vi "Clock Array to Clock Map.vi"(8 "error in (no error)":errorcluster, 10 "Clock Conversion Array":T3[](array[typedef]), 11 "Clock Convert Map in":T1) -> (0 "error out":errorcluster, 3 "Clock Convert Map out":T1)   [LabVIEW 2021, in "CIFClocks.lvlib"]
uses:
  CIFClocks.lvlib
  Typedef/Clock Conversion Map.ctl
  Typedef/Timestamp Pair.ctl
  Typedef/Clock Conversion.ctl
  <vilib>/Utility/miscctls.llb/LVMapReplaceAction.ctl
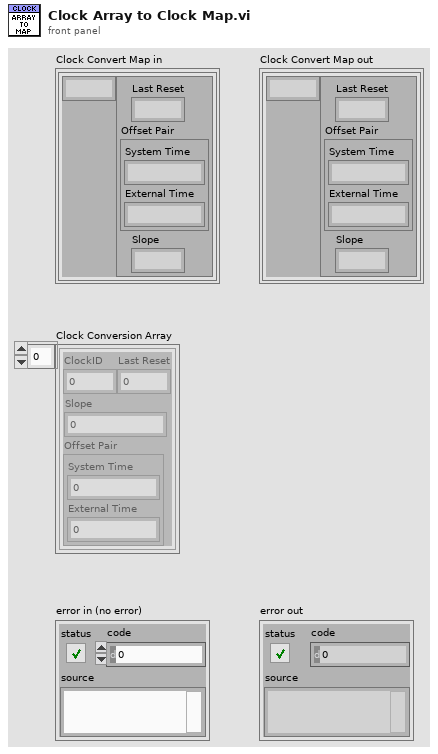
[diagram p1: front panel]
types:
  T1 = typedef "CIFClocks.lvlib/Clock Conversion Map.ctl" = map{u8, cluster{"Last Reset":u64, "Offset Pair":T2, "Slope":dbl}}
  T2 = typedef "CIFClocks.lvlib/Timestamp Pair.ctl" = cluster{"System Time":i64, "External Time":i64}
  T3 = typedef "CIFClocks.lvlib/Clock Conversion.ctl" = cluster{"ClockID":u8, "Last Reset":u64, "Offset Pair":T2, "Slope":dbl}
  T4 = typedef "LVMapReplaceAction.ctl" = enum32{"Modify Entry only if found", "Add or Modify Entry", "Delete Entry"}
  T5 = cluster{"Last Reset":u64, "Offset Pair":T2, "Slope":dbl}
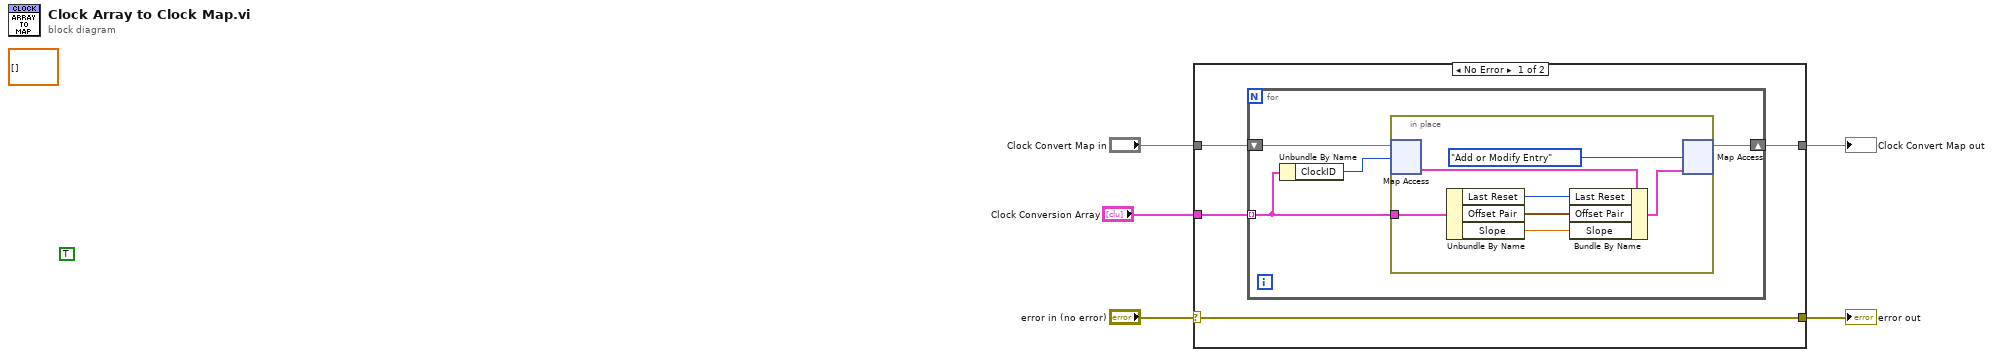
[diagram p0: block diagram]
diagram:
  (unwired) TRUE
  (unwired) dbl[][] []
  n1 = case shown="No Error" "error in (no error)" {
    selector: "error in (no error)" -> [w9 w22]
    tunnel: "Clock Convert Map in" -> [w8 w21]
    tunnel: [w9 w22] -> w3
    tunnel: "Clock Conversion Array" -> [w7 _]
    tunnel: [w6 w21] -> w1
    frame No Error {
      n2 = for {
        shift-right: [w10] -> w6
        shift-left: w8 -> [w13]
        tunnel: w7 -> [w11] mode=indexing
        n3 = Unbundle By Name(w11) -> ("ClockID"=w12:u8)
        n4 = in-place {
          in-place-border: w11 -> [w19]
          n5 = in-place-map #1(w13, w12) -> (w20:T5)  [unwired: 1 in, 1 out]
          n6 = Unbundle By Name(w19) -> ("Last Reset"=w18:u64, "Offset Pair"=w17:T2, "Slope"=w16:dbl)
          n7 = Bundle By Name(cluster=w20, "Last Reset"=w18, "Offset Pair"=w17, "Slope"=w16) -> (w15:T5)
          n8 = in-place-map #1(w15, LVMapReplaceAction."Add or Modify Entry" ("action")) -> (w10:T1)  [unwired: 2 out]
        }
      }
    }
    frame Error {
    }
  }
  "error out" <- w3
  "Clock Convert Map out" <- w1
